vi "ControlsToCommands.vi"(11 "input cluster":T1) -> (3 "output cluster":T2)   [LabVIEW 2016]
uses:
  ControlsToCommands.ctl
  Controls.ctl
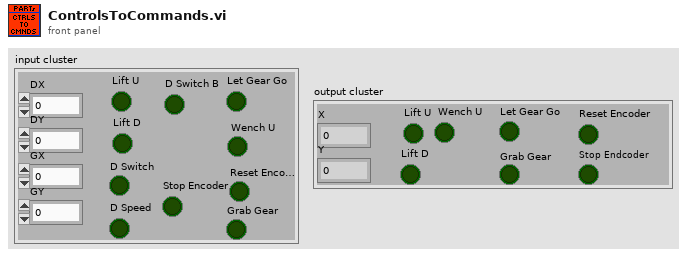
[diagram p1: front panel]
types:
  T1 = typedef "Controls.ctl" = cluster{"DX":dbl, "DY":dbl, "GX":dbl, "GY":dbl, "Lift U":bool, "D Switch":bool, "D Speed":bool, "D Switch B":bool, " Wench U":bool, "Lift D":bool, "Let Gear Go":bool, "Grab Gear":bool, "Reset Encoder":bool, "Stop Encoder":bool}
  T2 = typedef "ControlsToCommands.ctl" = cluster{"X":dbl, "Y":dbl, "Lift U":bool, " Wench U":bool, "Lift D":bool, "Let Gear Go":bool, "Grab Gear":bool, "Reset Encoder":bool, "Stop Endcoder":bool}
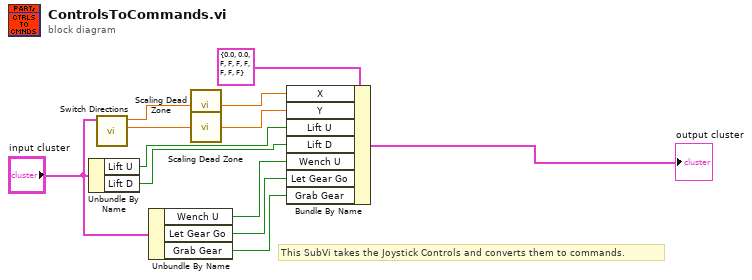
[diagram p0: block diagram]
diagram:
  # "This SubVi takes the Joystick Controls and converts them to commands."
  n1 = Unbundle By Name("input cluster") -> ("Lift U"=w8:bool, "Lift D"=w7:bool)
  n2 = call "Switch Directions.vi"("input cluster"="input cluster") -> ("Yout"=w1:dbl, "Xout"=w2:dbl)  [unwired: 9 in]
  n3 = Unbundle By Name("input cluster") -> ("Wench U"=w6:bool, "Let Gear Go"=w5:bool, "Grab Gear"=w4:bool)
  n4 = call "Scaling Dead Zone.vi"("Input"=w2) -> ("Output"=w10:dbl)  [unwired: 4 in]
  n5 = call "Scaling Dead Zone.vi"("Input"=w1) -> ("Output"=w11:dbl)  [unwired: 4 in]
  n6 = Bundle By Name(cluster=T2 {"X"=0.0, "Y"=0.0, "Lift U"=FALSE, " Wench U"=FALSE, "Lift D"=FALSE, "Let Gear Go"=FALSE, "Grab Gear"=FALSE, "Reset Encoder"=FALSE, "Stop Endcoder"=FALSE} ("input cluster"), "X"=w10, "Y"=w11, "Lift U"=w8, "Lift D"=w7, "Wench U"=w6, "Let Gear Go"=w5, "Grab Gear"=w4) -> (→"output cluster":T2)
